vi "Construct PLC.vi"(6 "MB Data Block (default)":refnum<data-value>, 7 "TCP Config":T1={"IP Address"="", "Port"=0, "Slave ID"=-1, "Timeout"=10000} {"Slave ID" format="%.0x"}, 8 "error in (no error)":errorcluster, 9 "PLC Config":T3={"Use TCP"=FALSE, "Reference Format"=6, "Swap Words"=FALSE, "Poll List"=[]} {"Reference Format" items=["4 Digits"=4, "5 Digits"=5, "6 Digits"=6]}, 10 "Serial Config":T2={"COM Port"="COM1", "Slave ID"=1, "baud rate (bps)"=460800, "Mode"=enum."RTU", "Parity"=0, "Flow Control"=0, "Timeout"=200, "Retries"=1, "Stop Bits"=10} {"Stop Bits" items=["1.0"=10, "1.5"=15, "2.0"=20]; "Flow Control" items=["None", "XON/XOFF", "RTS/CTS", "XON/XOFF & RTS/CTS", "DTR/DSR", "XON/XOFF & DTR/DSR"]; "Parity" items=["None", "Odd", "Even", "Mark", "Space"]}, 11 "PLC in":refnum<class "MB PLC Client.lvclass">) -> (0 "error out":errorcluster, 3 "PLC out":refnum<class "MB PLC Client.lvclass">)   [LabVIEW 2018, in "MB PLC Client.lvlib" / "MB PLC Client.lvclass"]
uses:
  MB PLC Client.lvclass
  Types/PLC Config_Cluster.ctl
  Types/MB Ref Range_Cluster.ctl
  Types/Serial Config_Cluster.ctl
  Types/TCP Config_Cluster.ctl
  Data/MB Data Block.lvclass
  MB PLC Client.lvclass/MB PLC Client.ctl
  MB PLC Client.lvlib
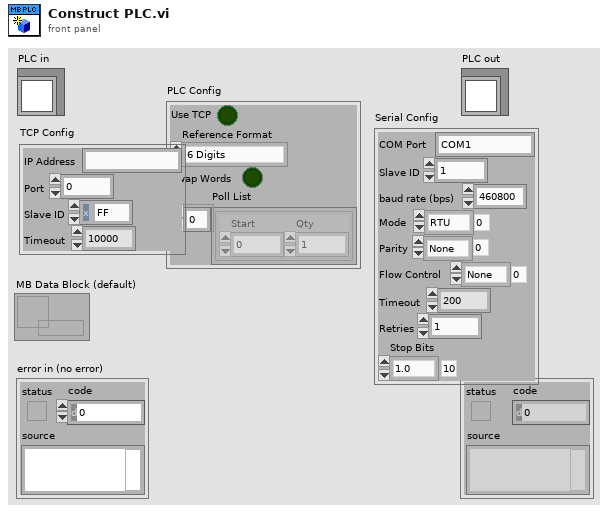
[diagram p1: front panel]
types:
  T1 = typedef "MB PLC Client.lvlib/TCP Config_Cluster.ctl" = cluster{"IP Address":string, "Port":u16, "Slave ID":i8, "Timeout":i32}
  T2 = typedef "MB PLC Client.lvlib/Serial Config_Cluster.ctl" = cluster{"COM Port":string, "Slave ID":u8, "baud rate (bps)":u32, "Mode":enum16{"RTU", "ASCII"}, "Parity":u16, "Flow Control":u16, "Timeout":u32, "Retries":u8, "Stop Bits":u16}
  T3 = typedef "MB PLC Client.lvlib/PLC Config_Cluster.ctl" = cluster{"Use TCP":bool, "Reference Format":u16, "Swap Words":bool, "Poll List":T4[]}
  T4 = typedef "MB PLC Client.lvlib/MB Ref Range_Cluster.ctl" = cluster{"Start":u32, "Qty":u16}
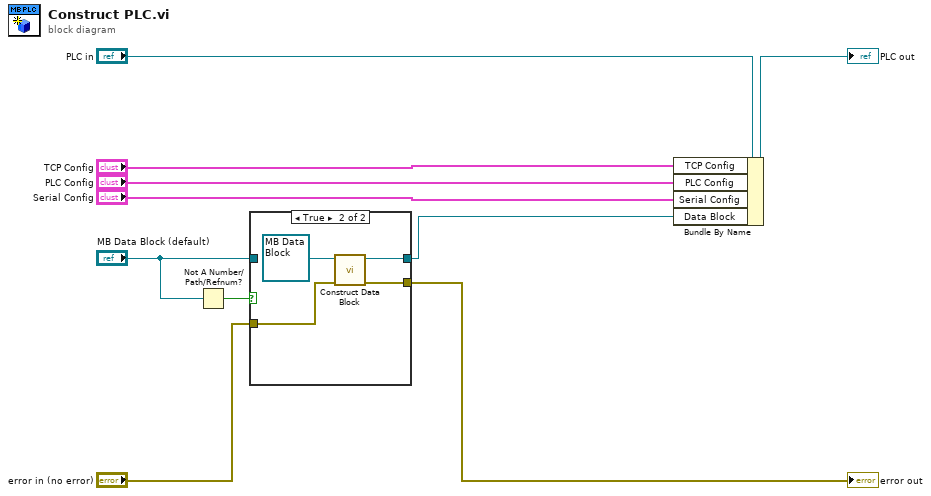
[diagram p0: block diagram]
diagram:
  n1 = Not A Number/Path/Refnum?(number/path/refnum="MB Data Block (default)") -> (NaN/Path/Refnum?=w5:bool)
  n2 = case shown="True" w5 {
    tunnel: "MB Data Block (default)" -> [w12 _]
    tunnel: [w12 w15] -> w1
    tunnel: "error in (no error)" -> [w11 w14]
    tunnel: [w11 w13] -> w2
    frame False {
    }
    frame True {
      n3 = call-dynamic "Construct Data Block.vi"("error in (no error)"=w14, "Modbus Data Store in"=refnum<class "MB Data Block.lvclass"> refnum) -> ("error out"=w13:errorcluster, "Cache Ref out"=w15:refnum<data-value>)  [unwired: 8 in]
    }
  }
  "error out" <- w2
  n4 = Bundle By Name(cluster="PLC in", "TCP Config"="TCP Config", "PLC Config"="PLC Config", "Serial Config"="Serial Config", "Data Block"=w1) -> (→"PLC out":refnum<class "MB PLC Client.lvclass">)
